vi "Track Object.vi"() -> ()   [LabVIEW 2012]
panel:
  in  "stop":bool
  out "Image":T1(plugin-control)
  out "Image 2":T1(plugin-control)
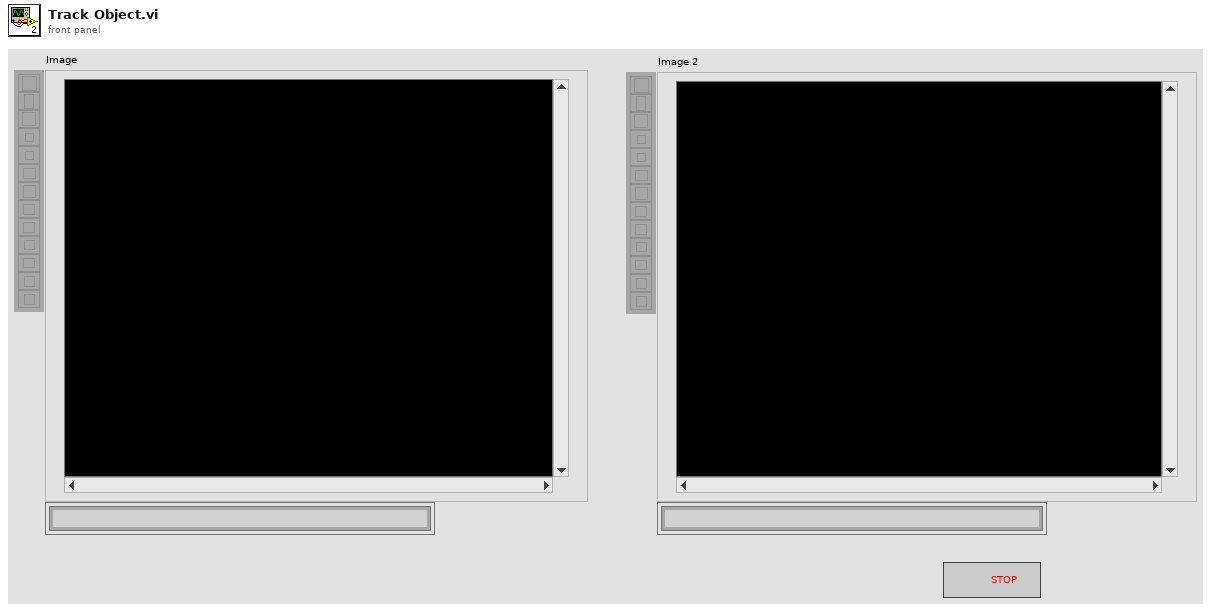
[diagram p1: front panel]
types:
  T1 = typedef "IMAQ Image.ctl" = refnum<image>
  T2 = cluster{"Global Rectangle":cluster{"x1Left":i32, "y1Top":i32, "x2Right":i32, "y2Bottom":i32}, "Centroid":cluster{"x":sgl, "y":sgl}, "Object Size":u32, "Score":dbl}[]
  T3 = cluster{"Shape Report (Shape Matching 1)[0]":cluster{"Global Rectangle":cluster{"x1Left":i32, "y1Top":i32, "x2Right":i32, "y2Bottom":i32}, "Centroid":cluster{"x":sgl, "y":sgl}, "Object Size":u32, "Score":dbl}, "Shape Report (Shape Matching 1)[1]":cluster{"Global Rectangle":cluster{"x1Left":i32, "y1Top":i32, "x2Right":i32, "y2Bottom":i32}, "Centroid":cluster{"x":sgl, "y":sgl}, "Object Size":u32, "Score":dbl}, "Shape Report (Shape Matching 1)[2]":cluster{"Global Rectangle":cluster{"x1Left":i32, "y1Top":i32, "x2Right":i32, "y2Bottom":i32}, "Centroid":cluster{"x":sgl, "y":sgl}, "Object Size":u32, "Score":dbl}, "Shape Report (Shape Matching 1)[3]":cluster{"Global Rectangle":cluster{"x1Left":i32, "y1Top":i32, "x2Right":i32, "y2Bottom":i32}, "Centroid":cluster{"x":sgl, "y":sgl}, "Object Size":u32, "Score":dbl}, "Shape Report (Shape Matching 1)[4]":cluster{"Global Rectangle":cluster{"x1Left":i32, "y1Top":i32, "x2Right":i32, "y2Bottom":i32}, "Centroid":cluster{"x":sgl, "y":sgl}, "Object Size":u32, "Score":dbl}, "Shape Report (Shape Matching 1)[5]":cluster{"Global Rectangle":cluster{"x1Left":i32, "y1Top":i32, "x2Right":i32, "y2Bottom":i32}, "Centroid":cluster{"x":sgl, "y":sgl}, "Object Size":u32, "Score":dbl}, "Shape Report (Shape Matching 1)[6]":cluster{"Global Rectangle":cluster{"x1Left":i32, "y1Top":i32, "x2Right":i32, "y2Bottom":i32}, "Centroid":cluster{"x":sgl, "y":sgl}, "Object Size":u32, "Score":dbl}, "Shape Report (Shape Matching 1)[7]":cluster{"Global Rectangle":cluster{"x1Left":i32, "y1Top":i32, "x2Right":i32, "y2Bottom":i32}, "Centroid":cluster{"x":sgl, "y":sgl}, "Object Size":u32, "Score":dbl}, "Shape Report (Shape Matching 1)[8]":cluster{"Global Rectangle":cluster{"x1Left":i32, "y1Top":i32, "x2Right":i32, "y2Bottom":i32}, "Centroid":cluster{"x":sgl, "y":sgl}, "Object Size":u32, "Score":dbl}}
  T4 = cluster{"x1Left":i32, "y1Top":i32, "x2Right":i32, "y2Bottom":i32}
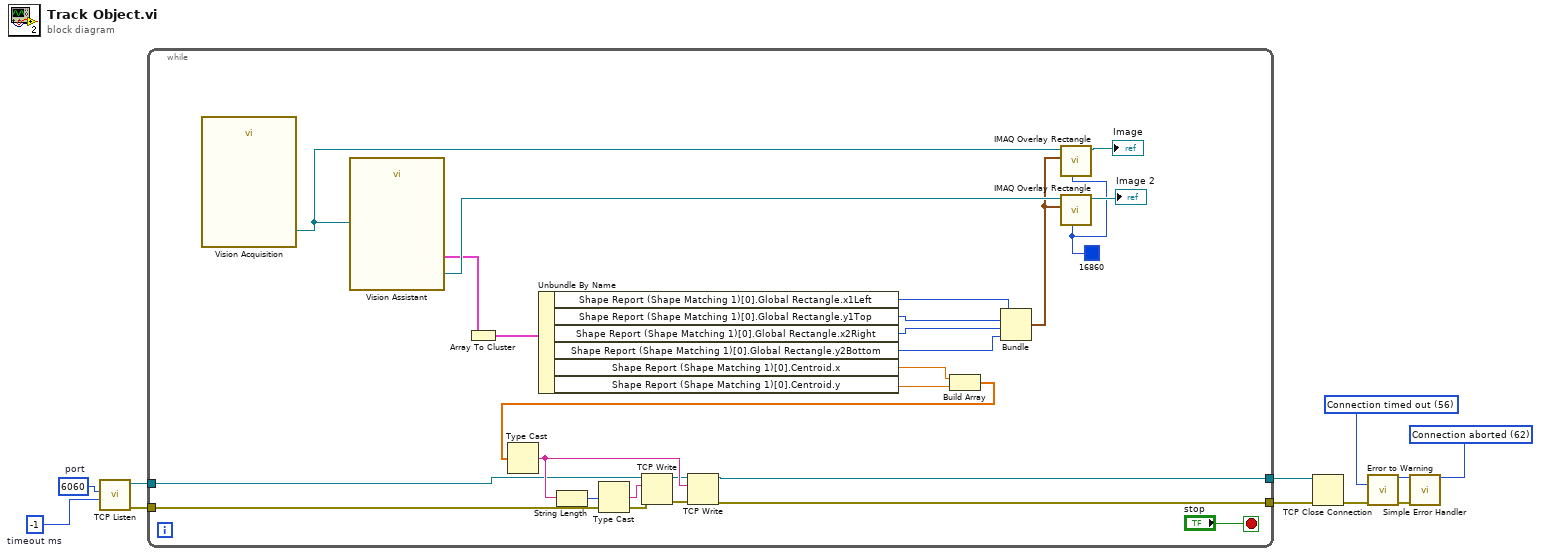
[diagram p0: block diagram]
diagram:
  w4 = 56 items=["No Error", "Argument Error", "Memory Full", "Out of Zone", "End of File", "File Already Open", "Generic File IO Error", "File Not Found", "File Permission Error", "Disk Full", "Duplicate Path", "Too Many Files Open", "Not Enabled", "Resource File Not Found", "Cannot Add Resource", "Resource Not Found", "Image Not Found", "Image Memory Error", "Pen Does Not Exist", "Config Bad Type", "Config Token Not Found", "Config Parse Error", "Config Memory Error", "Bad External Code Format", "Bad External Code Offset", "External Code Not Present", "Null Window", "Destroy Window Mixup", "Null Menu", "Print Aborted", "Bad Print Record", "Print Driver Error", "Windows Error During Print", "Memory Error During Print", "Print Dialog Error", "Generic Print Error", "Invalid Device Refnum", "Device Not Found", "Device Parameter Error", "Device Unit Error", "Can't Open Device", "Device Call Aborted", "Generic Error", "Cancelled By User", "Object ID Too Low", "Object ID Too High", "Object Not In Heap", "Unknown Heap", "Bad DefProc ID", "DefProc Not In Table", "Message Out Of Range", "Null Method", "Unknown Message", "Manager Call Not Supported", "Bad address", "Connection In progress", "Connection timed out", "Connection is already in progress", "Network attribute not supported", "Network error", "Address in use", "System out of memory", "Connection aborted", "Connection refused", "Connection is not connected", "Connection is already connected", "Connection closed", "Initialize error (interapplication manager)", "Bad occurrence", "Wait on unbound occurrence handler", "Occurrence queue overflow", "Bad path", "Semaphore not signaled", "Unrecognized type (interapplication manager)"] ("2nd Error to Convert")
  w5 = 62 items=["No Error", "Argument Error", "Memory Full", "Out of Zone", "End of File", "File Already Open", "Generic File IO Error", "File Not Found", "File Permission Error", "Disk Full", "Duplicate Path", "Too Many Files Open", "Not Enabled", "Resource File Not Found", "Cannot Add Resource", "Resource Not Found", "Image Not Found", "Image Memory Error", "Pen Does Not Exist", "Config Bad Type", "Config Token Not Found", "Config Parse Error", "Config Memory Error", "Bad External Code Format", "Bad External Code Offset", "External Code Not Present", "Null Window", "Destroy Window Mixup", "Null Menu", "Print Aborted", "Bad Print Record", "Print Driver Error", "Windows Error During Print", "Memory Error During Print", "Print Dialog Error", "Generic Print Error", "Invalid Device Refnum", "Device Not Found", "Device Parameter Error", "Device Unit Error", "Can't Open Device", "Device Call Aborted", "Generic Error", "Cancelled By User", "Object ID Too Low", "Object ID Too High", "Object Not In Heap", "Unknown Heap", "Bad DefProc ID", "DefProc Not In Table", "Message Out Of Range", "Null Method", "Unknown Message", "Manager Call Not Supported", "Bad address", "Connection In progress", "Connection timed out", "Connection is already in progress", "Network attribute not supported", "Network error", "Address in use", "System out of memory", "Connection aborted", "Connection refused", "Connection is not connected", "Connection is already connected", "Connection closed", "Initialize error (interapplication manager)", "Bad occurrence", "Wait on unbound occurrence handler", "Occurrence queue overflow", "Bad path", "Semaphore not signaled", "Unrecognized type (interapplication manager)"] ("1st Error to Convert")
  w9 = u16 6060  # port
  w10 = -1  # timeout ms
  n1 = call <vilib>:"TCP Listen.vi"("timeout ms (wait forever: -1)"=w10, "port"=w9) -> ("error out"=w1:errorcluster, "connection ID"=w8:refnum<k5>)  [unwired: 5 in, 3 out]
  n2 = while {
    tunnel: w8 -> [w17]
    tunnel: [w16] -> w3
    tunnel: [w15] -> w2
    tunnel: w1 -> [w14]
    stop <- "stop" stop-if-true
    w24 = u32 16860 ("Color")
    n3 = call "Vision Acquisition"() -> ("Image Out"=w33:T1)  [unwired: 25 in, 2 out]
    n4 = call "Vision Assistant"("Image In"=w33) -> ("Image Out"=w32:T1, "Shape Report (Shape Matching 1)"=w29:T2)  [unwired: 23 in, 2 out]
    n5 = Array To Cluster(array=w29) -> (cluster=w34:T3)
    n6 = Unbundle By Name(w34) -> ("Shape Report (Shape Matching 1)[0].Global Rectangle.x1Left"=w28:i32, "Shape Report (Shape Matching 1)[0].Global Rectangle.y1Top"=w27:i32, "Shape Report (Shape Matching 1)[0].Global Rectangle.x2Right"=w26:i32, "Shape Report (Shape Matching 1)[0].Global Rectangle.y2Bottom"=w25:i32, "Shape Report (Shape Matching 1)[0].Centroid.x"=w13:sgl, "Shape Report (Shape Matching 1)[0].Centroid.y"=w12:sgl)
    n7 = Build Array(w13, w12) -> (w11:sgl[])
    n8 = Type Cast(x=w11) -> (*(type *) &x=w22:string)  [unwired: 1 in]
    n9 = String Length(string=w22) -> (length=w20:i32)
    n10 = Type Cast(x=w20) -> (*(type *) &x=w21:string)  [unwired: 1 in]
    n11 = TCP Write(connection ID=w17, data in=w21, error in (no error)=w14) -> (connection ID out=w18:refnum<k5>, error out=w19:errorcluster)  [unwired: 1 in, 1 out]
    n12 = TCP Write(connection ID=w18, data in=w22, error in (no error)=w19) -> (connection ID out=w16:refnum<k5>, error out=w15:errorcluster)  [unwired: 1 in, 1 out]
    n13 = Bundle("x1Left"=w28, "y1Top"=w27, "x2Right"=w26, "y2Bottom"=w25) -> (w23:T4)  [unwired: 1 in]
    n14 = call "IMAQ Overlay Rectangle"("Color"=w24, "Rectangle"=w23, "Image"=w33) -> ("Image Out"=→"Image":T1)  [unwired: 7 in, 1 out]
    n15 = call "IMAQ Overlay Rectangle"("Color"=w24, "Rectangle"=w23, "Image"=w32) -> ("Image Out"=→"Image 2":T1)  [unwired: 7 in, 1 out]
  }
  n16 = TCP Close Connection(connection ID=w3, error in (no error)=w2) -> (error out=w7:errorcluster)  [unwired: 1 in, 1 out]
  n17 = call <vilib>:"Error to Warning.vi"("1st Error to Convert"=w5, "2nd Error to Convert"=w4, "error in"=w7) -> ("warning out"=w6:errorcluster)  [unwired: 12 in]
  n18 = call <vilib>:"Simple Error Handler.vi"("error in (no error)"=w6) -> ()  [unwired: 4 in, 5 out]
